vi "F Term.vi"(7 "Output Range":T1={"Min"=-50.0, "Max"=50.0}, 9 "Setpoint":dbl, 10 "F Gain":dbl) -> (2 "Output":dbl, 5 "Remaining Range":T1={"Min"=-50.0, "Max"=50.0})   [LabVIEW 2020, in "IG PID.lvlib" / "PID.lvclass"]
uses:
  PID.lvclass
  Output Range.ctl
  IG PID.lvlib
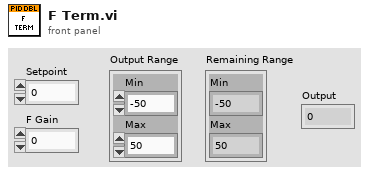
[diagram p1: front panel]
types:
  T1 = typedef "IG PID.lvlib/Output Range.ctl" = cluster{"Min":dbl, "Max":dbl}
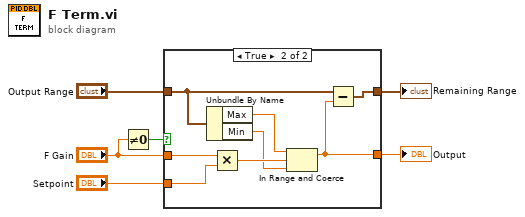
[diagram p0: block diagram]
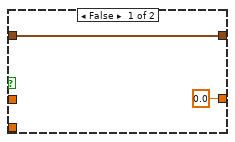
[diagram p2: hidden frame]
diagram:
  n1 = Not Equal To 0?(x="F Gain") -> (x != 0?=w1:bool)
  n2 = case shown="True" w1 {
    tunnel: "Setpoint" -> [_ w16]
    tunnel: "Output Range" -> [w8 w12]
    tunnel: [0.0 ("Max") w11] -> w4
    tunnel: [w8 w10] -> w3
    tunnel: "F Gain" -> [_ w9]
    frame False {
    }
    frame True {
      n3 = Unbundle By Name(w12) -> ("Max"=w13:dbl, "Min"=w14:dbl)
      n4 = Multiply(x=w9, y=w16) -> (x*y=w15:dbl)
      n5 = In Range and Coerce(upper limit=w13, x=w15, lower limit=w14) -> (coerced(x)=w11:dbl)  [unwired: 1 out]
      n6 = Subtract(x=w12, y=w11) -> (x-y=w10:T1)
    }
  }
  "Output" <- w4
  "Remaining Range" <- w3
